vi "Helper Action.vi"(8 "error in (no error)":errorcluster, 9 "Message Data":variant, 10 "Message":string, 11 "Mock Process In":refnum<class "Mock Process.lvclass">) -> (0 "error out":errorcluster, 2 "Loop Period [ms]":i32=-1, 3 "Mock Process Out":refnum<class "Mock Process.lvclass">)   [LabVIEW 2020, in "Mock Process.lvclass"]
uses:
  Mock Process.lvclass
  Mock Process.lvclass/Mock Process.ctl
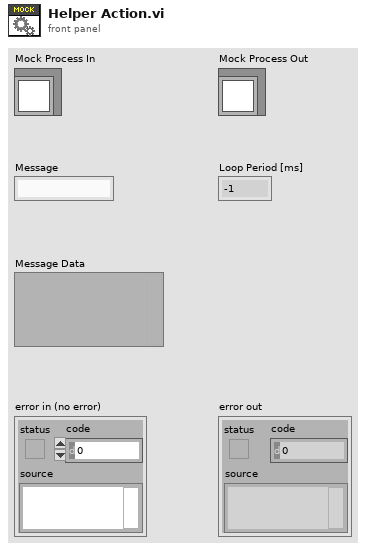
[diagram p1: front panel]
types:
  T1 = cluster{"Message":string, "Message Data":variant}
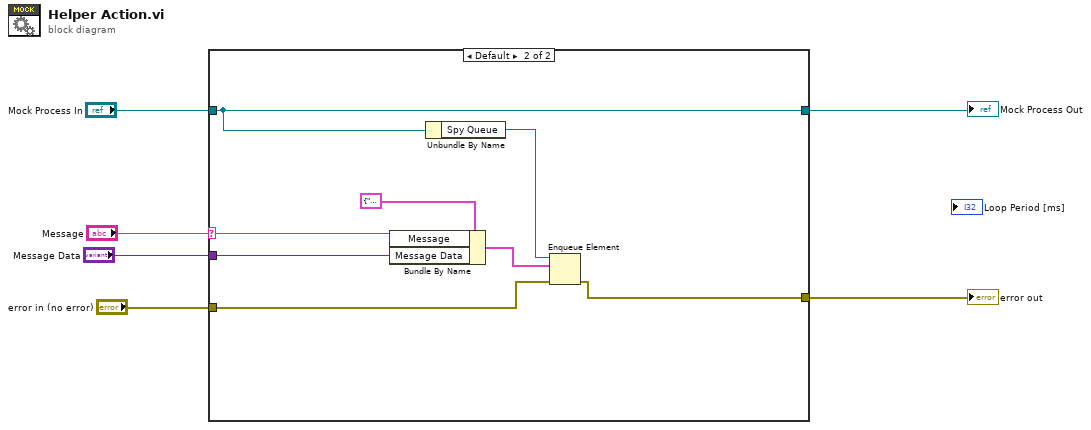
[diagram p0: block diagram]
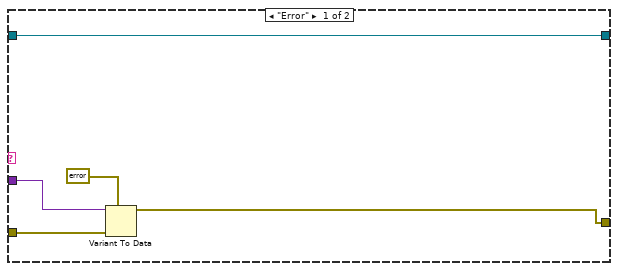
[diagram p2: hidden frame]
diagram:
  n1 = case shown="Default" "Message" {
    selector: "Message" -> [_ w14]
    tunnel: "Mock Process In" -> [w7 w12]
    tunnel: [w9 w16] -> w5
    tunnel: "error in (no error)" -> [w10 w15]
    tunnel: "Message Data" -> [w11 w13]
    tunnel: [w7 w12] -> w1
    frame "Error" {
      n2 = Variant To Data(error in=w10, type=errorcluster {"status"=FALSE, "code"=0, "source"=""} ("error out"), Variant=w11) -> (data=w9:errorcluster)  [unwired: 1 out]
    }
    frame Default {
      n3 = Bundle By Name(cluster=T1 {"Message"="", "Message Data"=variant} ("Message Cluster"), "Message"=w14, "Message Data"=w13) -> (w19:T1)
      n4 = Unbundle By Name(w12) -> ("Spy Queue"=w18:refnum<queue>)
      n5 = Enqueue Element(queue=w18, element=w19, error in (no error)=w15) -> (error out=w16:errorcluster)  [unwired: 1 in, 2 out]
    }
  }
  "error out" <- w5
  "Mock Process Out" <- w1
